vi "test.vi"() -> ()   [LabVIEW 2011]
uses:
  CH368_PY_LIB.dll
  CH368_PY.dll
panel:
  out "DrvVersion":u32
  out "Version":u32
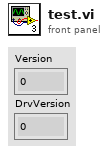
[diagram p1: front panel]
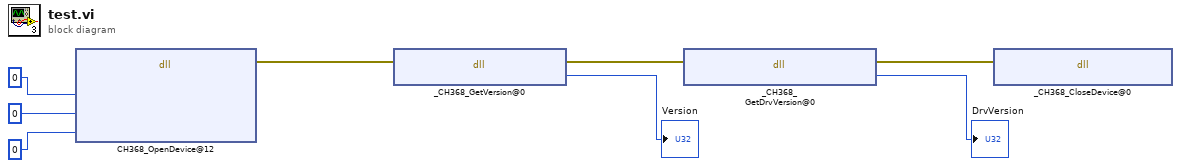
[diagram p0: block diagram]
diagram:
  n1 = dll-call lib="E:/_pan_file/_my_nut/CH368_PY_LIB/CH368_PY_mingw/CH368_PY.dll" fn="CH368_OpenDevice@12"("iEnableMemory"=0, "iEnableInterrupt"=0, "iInterruptMode"=u8 0) -> (error out=w7:errorcluster)  [unwired: 7 in, 1 out]
  n2 = dll-call lib="E:/_pan_file/_my_nut/CH368_PY_LIB/CH368_PY_mingw/CH368_PY_LIB.dll" fn="_CH368_GetVersion@0"(error in=w7) -> (error out=w3:errorcluster, "Version"=→"Version":u32)  [unwired: 2 in, 1 out]
  n3 = dll-call lib="E:/_pan_file/_my_nut/CH368_PY_LIB/CH368_PY_mingw/CH368_PY_LIB.dll" fn="_CH368_GetDrvVersion@0"(error in=w3) -> (error out=w2:errorcluster, "DrvVersion"=→"DrvVersion":u32)  [unwired: 2 in, 1 out]
  n4 = dll-call lib="E:/_pan_file/_my_nut/CH368_PY_LIB/CH368_PY_mingw/CH368_PY_LIB.dll" fn="_CH368_CloseDevice@0"(error in=w2) -> ()  [unwired: 3 in, 2 out]
